vi "r2_maker.vi"(0 "yr":dbl[](array[numeric]), 1 "in":dbl[](array[numeric]), 2 "b2":dbl[](array[numeric]), 3 "N":i32, 4 "xr":T1) -> (7 "r2":T1)   [LabVIEW 2014]
uses:
  <vilib>/Analysis/Matrix/Datatypes/RealMatrix.ctl
  <vilib>/Analysis/Matrix/Numeric/Conversions/Matrix To Array - RM.vi
  <vilib>/Analysis/Matrix/NI_Matrix.lvlib
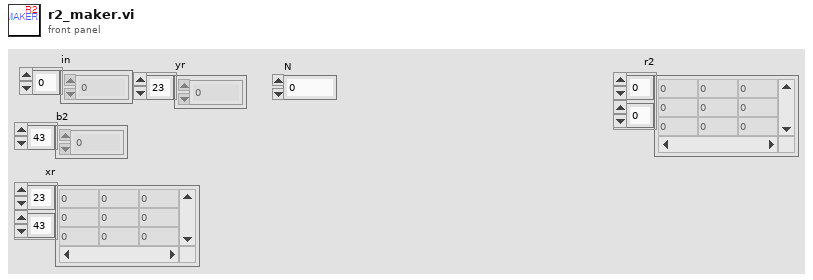
[diagram p1: front panel]
types:
  T1 = typedef "NI_Matrix.lvlib/RealMatrix.ctl" = dbl[][]
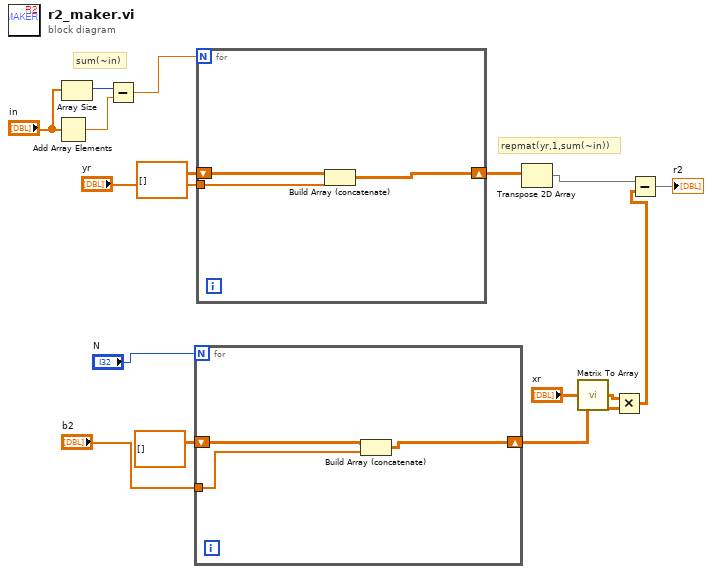
[diagram p0: block diagram]
diagram:
  # "sum(~in)"
  # "repmat(yr,1,sum(~in))"
  n1 = Add Array Elements(numeric array="in") -> (sum=w11:dbl)
  n2 = Array Size(array="in") -> (size(s)=w12:i32)
  n3 = Subtract(x=w12, y=w11) -> (x-y=w10:dbl)
  n4 = for {
    N: "N" -> [_]
    shift-right: [w18] -> w5
    shift-left: dbl[][] [] -> [w19]
    tunnel: "b2" -> [w17]
    n5 = Build Array (concatenate)(w19, w17) -> (w18:dbl[][])
  }
  n6 = for {
    N: w10 -> [_]
    tunnel: "yr" -> [w22]
    shift-right: [w21] -> w14
    shift-left: dbl[][] [] -> [w20]
    n7 = Build Array (concatenate)(w20, w22) -> (w21:dbl[][])
  }
  n8 = Transpose 2D Array(2D array=w14) -> (transposed array=w4:dbl[][])
  n9 = call-poly <vilib>:"Matrix To Array.vi"("Real Matrix"="xr") -> ("Real 2D Array"=w1:dbl[][])
  n10 = Multiply ("Multiply.vi")(x=w1, y=w5) -> (x*y=w3:dbl[][])
  n11 = Subtract ("Subtract.vi")(x=w4, y=w3) -> (x-y=→"r2":dbl[][])
